vi "Sequence.CreateSteps.vi"(7 "Step":T3, 8 "error in (no error)":errorcluster, 9 "StepInfo":T2, 10 "Iteration":i32, 11 "Refs":T1) -> (0 "error out":errorcluster, 3 "Refs out":T1)   [LabVIEW 2013, in "Simple Sequence Editor.lvlib"]
uses:
  Simple Sequence Editor.lvlib
  Types/Sequence.MainSeqRefs.ctl
  NationalInstruments.VeriStand.RealTimeSequenceDefinitionApi
  Types/Compiled.StepProperties.ctl
  Types/Compiled.IOStateProperties.ctl
  Types/Compiled.StepElementProperties.ctl
  Types/ChannelProperties.ctl
  Types/StepTypes.ctl
  Types/Compiled.StepCondition.ctl
  Types/OperationTypes.ctl
  Constants.vi
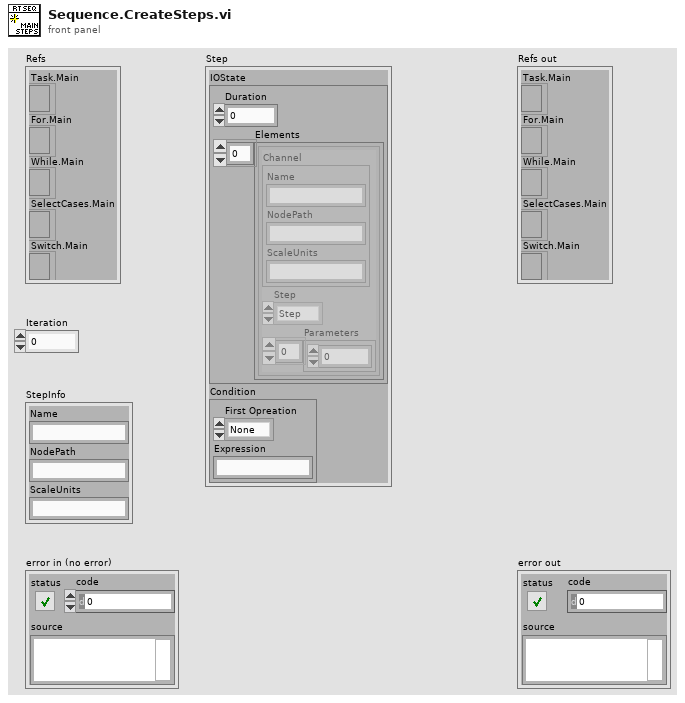
[diagram p1: front panel]
types:
  T1 = typedef "Simple Sequence Editor.lvlib/Sequence.MainSeqRefs.ctl" = cluster{"Task.Main":refnum<k24>, "For.Main":refnum<k24>, "While.Main":refnum<k24>, "SelectCases.Main":refnum<k24>, "Switch.Main":refnum<k24>}
  T2 = typedef "Simple Sequence Editor.lvlib/ChannelProperties.ctl" = cluster{"Name":string, "NodePath":string, "ScaleUnits":string}
  T3 = typedef "Simple Sequence Editor.lvlib/Compiled.StepProperties.ctl" = cluster{"IOState":T4, "Condition":T7}
  T4 = typedef "Simple Sequence Editor.lvlib/Compiled.IOStateProperties.ctl" = cluster{"Duration":dbl, "Elements":T5[]}
  T5 = typedef "Simple Sequence Editor.lvlib/Compiled.StepElementProperties.ctl" = cluster{"Channel":T2, "Step":T6, "Parameters":dbl[]}
  T6 = typedef "Simple Sequence Editor.lvlib/StepTypes.ctl" = enum8{"Step", "iStep", "Ramp", "Unchanged", "Unknown"}
  T7 = typedef "Simple Sequence Editor.lvlib/Compiled.StepCondition.ctl" = cluster{"First Opreation":T8, "Expression":string}
  T8 = typedef "Simple Sequence Editor.lvlib/OperationTypes.ctl" = enum8{"None", "&&", "||"}
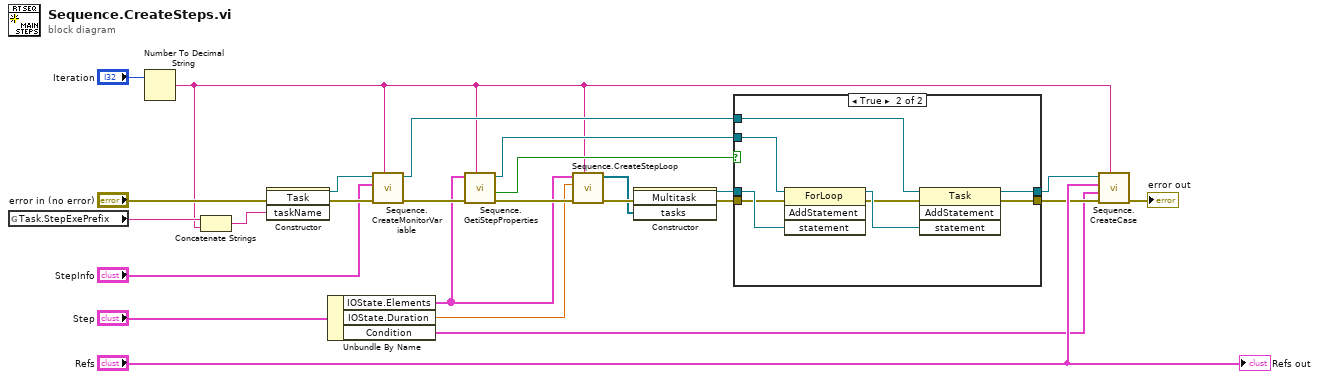
[diagram p0: block diagram]
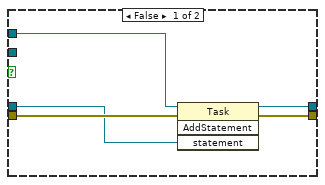
[diagram p2: hidden frame]
diagram:
  n1 = global read "Constants.vi" "Task.StepExePrefix"() -> (w25:string)
  n2 = Number To Decimal String(number="Iteration") -> (decimal integer string=w2:string)  [unwired: 1 in]
  n3 = Concatenate Strings(w25, w2) -> (w16:string)
  n4 = constructor class="Task"(error in="error in (no error)", "taskName"=w16) -> (reference out=w21:refnum<k24>, error out=w20:errorcluster)  [unwired: 2 in, 2 out]
  n5 = Unbundle By Name("Step") -> ("IOState.Elements"=w5:T5[], "IOState.Duration"=w4:dbl, "Condition"=w1:T7)
  n6 = call "Sequence.CreateMonitorVariable.vi"("Iteration"=w2, "error in (no error)"=w20, "StepInfo"="StepInfo", "Task Ref"=w21) -> ("error out"=w22:errorcluster, "Task Ref out"=w23:refnum<k24>)  [unwired: 6 in]
  n7 = call "Sequence.GetiStepProperties.vi"("Iteration"=w2, "error in (no error)"=w22, "Elements"=w5) -> ("error out"=w10:errorcluster, "Step Conatins iStep?"=w13:bool, "iStepForLoop Ref"=w3:refnum<k24>)  [unwired: 6 in]
  n8 = call "Sequence.CreateStepLoop.vi"("Iteration"=w2, "error in (no error)"=w10, "Duration"=w4, "Elements"=w5) -> ("error out"=w9:errorcluster, "Tasks"=w8:refnum<k24>[])  [unwired: 6 in]
  n9 = constructor class="Multitask"(error in=w9, "tasks"=w8) -> (reference out=w11:refnum<k24>, error out=w12:errorcluster)  [unwired: 2 in, 2 out]
  n10 = case shown="True" w13 {
    tunnel: w3 -> [_ w38]
    tunnel: w11 -> [w26 w37]
    tunnel: w12 -> [w29 w36]
    tunnel: [w28 w32] -> w14
    tunnel: [w27 w31] -> w15
    tunnel: w23 -> [w30 w35]
    frame False {
      n11 = invoke class="Task" method="AddStatement"(reference=w30, error in=w29, "statement"=w26) -> (reference out=w27:refnum<k24>, error out=w28:errorcluster)  [unwired: 1 in, 2 out]
    }
    frame True {
      n12 = invoke class="ForLoop" method="AddStatement"(reference=w38, error in=w36, "statement"=w37) -> (reference out=w34:refnum<k24>, error out=w33:errorcluster)  [unwired: 1 in, 2 out]
      n13 = invoke class="Task" method="AddStatement"(reference=w35, error in=w33, "statement"=w34) -> (reference out=w31:refnum<k24>, error out=w32:errorcluster)  [unwired: 1 in, 2 out]
    }
  }
  n14 = call "Sequence.CreateCase.vi"("Iteration"=w2, "error in (no error)"=w14, "Condition"=w1, "Refs"="Refs", "TaskRef"=w15) -> ("error out"=→"error out":errorcluster)  [unwired: 6 in]
  "Refs out" <- "Refs"
